vi "dfd_Interpolator Simu.vi"(11 "factor":i32) -> (3 "dup factor":i32)   [LabVIEW 2017, in "NI_DigFilter_FXP.lvlib"]
uses:
  <vilib>/addons/Digital Filter Design/NI_DigFilter_FXP.lvlib
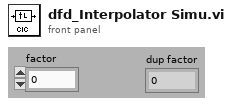
[diagram p1: front panel]
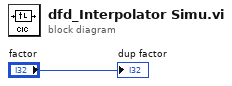
[diagram p0: block diagram]
diagram:
  "dup factor" <- "factor"
